vi "AM_DeModulationMaybe.vi"(4 "Fs":dbl, 6 "Fc":dbl, 10 "mod_signal":dbl[](array[numeric])) -> (2 "message":dbl[](array[numeric]))   [LabVIEW 2011]
uses:
  <vilib>/Analysis/3filter.llb/Equi-Ripple LowPass (DBL).vi
  <vilib>/Analysis/NI_AALBase.lvlib
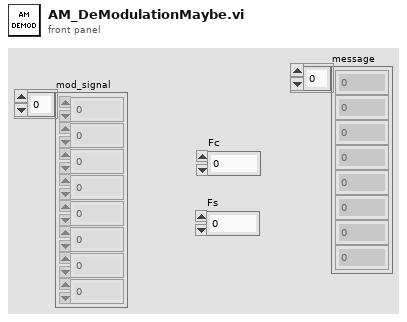
[diagram p1: front panel]
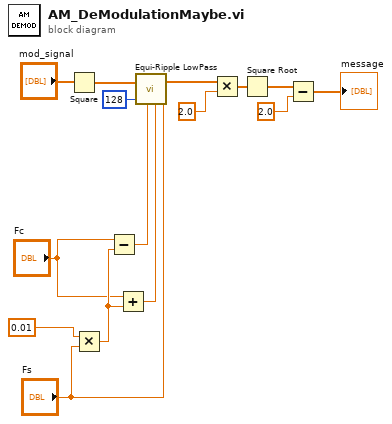
[diagram p0: block diagram]
diagram:
  n1 = Square(x="mod_signal") -> (x^2=w14:dbl[])
  n2 = Multiply(x=0.01, y="Fs") -> (x*y=w5:dbl)
  n3 = Subtract(x="Fc", y=w5) -> (x-y=w3:dbl)
  n4 = Add(x="Fc", y=w5) -> (x+y=w2:dbl)
  n5 = call-poly <vilib>:"Equi-Ripple LowPass.vi"("# of taps"=128, "pass freq"=w3, "stop freq"=w2, "sampling freq: fs"="Fs", "X"=w14) -> ("Filtered X"=w13:dbl[])  [unwired: 1 in, 1 out]
  n6 = Multiply(x=w13, y=2.0) -> (x*y=w11:dbl[])
  n7 = Square Root(x=w11) -> (sqrt(x)=w10:dbl[])
  n8 = Subtract(x=w10, y=2.0) -> (x-y=→"message":dbl[])
